vi "CH0_Move.vi"(6 "Direction":bool, 7 "Channel":u8, 8 "error in (no error)":errorcluster, 9 "CH0 Steps/deg":u16, 10 "Collection HWP Angle":dbl, 11 "MB_Master in":refnum<class "MB_Master.lvclass">) -> (0 "error out":errorcluster, 3 "MB_Master out":refnum<class "MB_Master.lvclass">)   [LabVIEW 2021]
uses:
  <vilib>/Plasmionique/MB Master/MB_Master/MB_Master.lvclass
  <vilib>/Plasmionique/MB Master/MB Master.lvlib
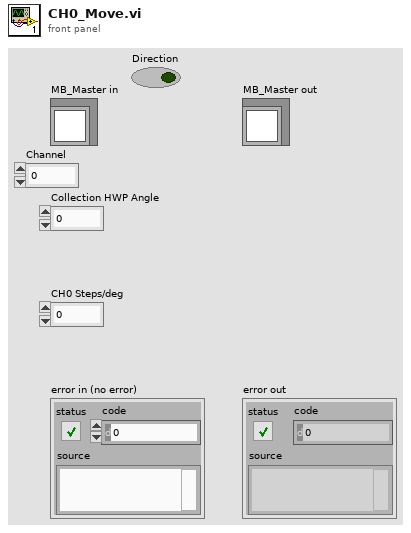
[diagram p1: front panel]
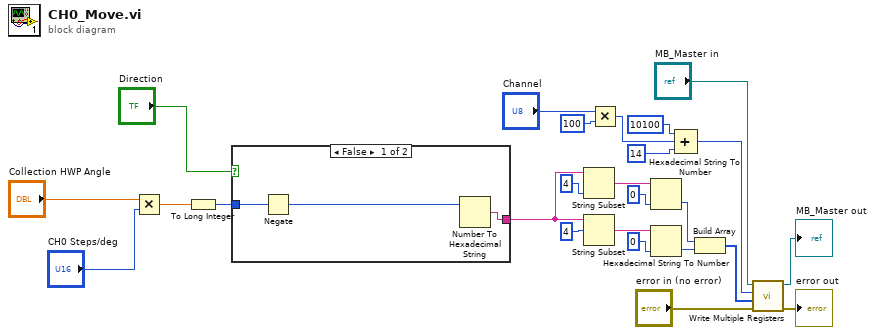
[diagram p0: block diagram]
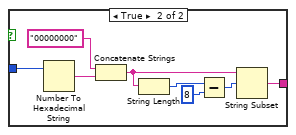
[diagram p2: hidden frame]
diagram:
  n1 = Multiply(x="Collection HWP Angle", y="CH0 Steps/deg") -> (x*y=w25:dbl)
  n2 = To Long Integer(number=w25) -> (32bit integer=w1:i32)
  n3 = case shown="False" "Direction" {
    tunnel: [w26 w31] -> w2
    tunnel: w1 -> [w27 w30]
    frame False {
      n4 = Negate(x=w27) -> (-x=w28:i32)
      n5 = Number To Hexadecimal String(2:w28) -> (0:w26:string)  [unwired: 1 in]
    }
    frame True {
      n6 = Number To Hexadecimal String(2:w30) -> (0:w29:string)  [unwired: 1 in]
      n7 = Concatenate Strings("00000000", w29) -> (w36:string)
      n8 = String Length(string=w36) -> (length=w35:i32)
      n9 = Subtract(x=w35, y=8) -> (x-y=w33:i32)
      n10 = String Subset(string=w36, offset (0)=w33) -> (substring=w31:string)  [unwired: 1 in]
    }
  }
  n11 = String Subset(string=w2, length (rest)=4 ("length (rest)")) -> (substring=w16:string)  [unwired: 1 in]
  n12 = String Subset(string=w2, offset (0)=4) -> (substring=w18:string)  [unwired: 1 in]
  n13 = Multiply(x="Channel", y=u16 100) -> (x*y=w9:u16)
  n14 = Hexadecimal String To Number(string=w16, default (0uL)=u16 0 ("default (0 U32)")) -> (number=w20:u16)  [unwired: 1 in, 1 out]
  n15 = Hexadecimal String To Number(string=w18, default (0uL)=u16 0 ("default (0 U32)")) -> (number=w21:u16)  [unwired: 1 in, 1 out]
  n16 = Compound Arithmetic op=ADD(u16 10100 ("value"), w9, u8 14 ("value")) -> (w4:u16)
  n17 = Build Array(w20, w21) -> (w11:u16[])
  n18 = call <vilib>:"Write Multiple Registers.vi"("error in (no error)"="error in (no error)", "values"=w11, "starting address"=w4, "MB session in"="MB_Master in") -> ("error out"=→"error out":errorcluster, "MB session out"=→"MB_Master out":refnum<class "MB_Master.lvclass">)  [unwired: 6 in]
